vi "ThermoRecDisplay.vi"() -> ()   [LabVIEW 2016]
panel:
  out "SW OPC Error":bool
  out "SS OPC Error":bool
  out "SW ThermoRec Information":string
  out "SS ThermoRec Information":string
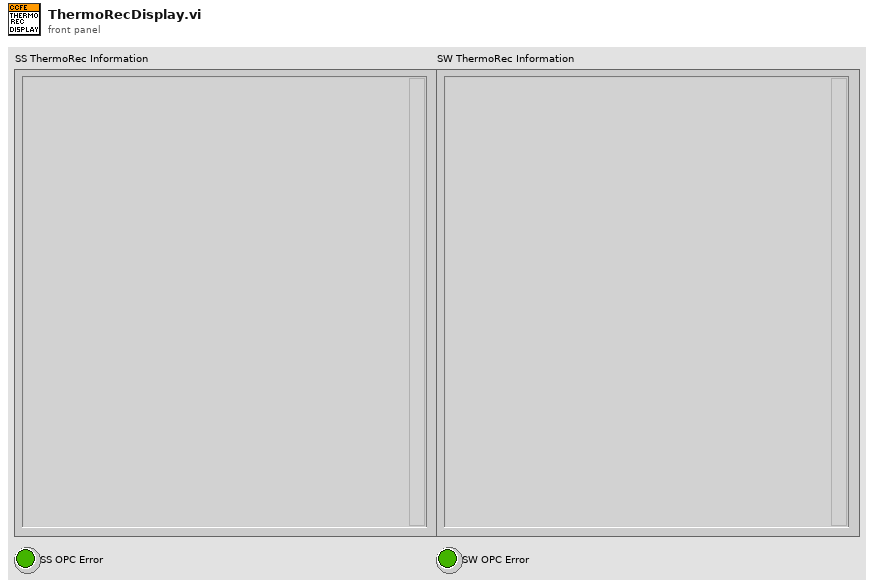
[diagram p1: front panel]
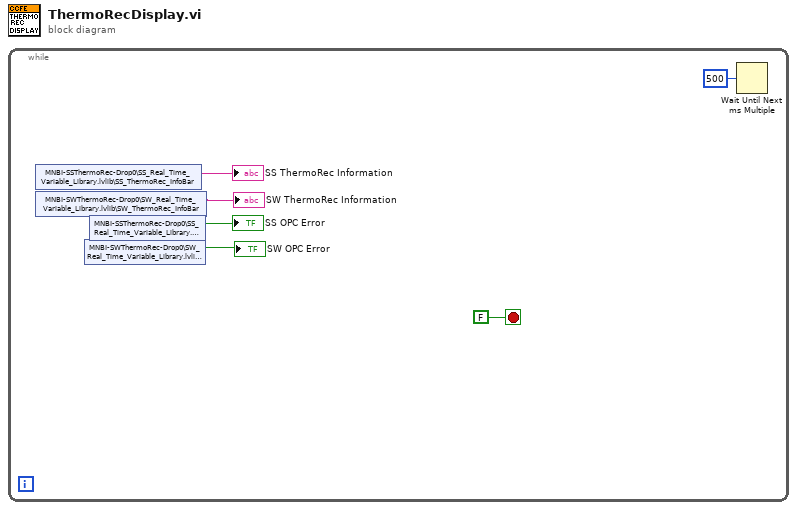
[diagram p0: block diagram]
diagram:
  n1 = while {
    stop <- FALSE stop-if-true
    n2 = shared-variable "MNBI-SSThermoRec-Drop0\\SS_Real_Time_Variable_Library.lvlib\\SS_ThermoRec_InfoBar"() -> (→"SS ThermoRec Information":string)  [unwired: 1 in, 1 out]
    n3 = shared-variable "MNBI-SWThermoRec-Drop0\\SW_Real_Time_Variable_Library.lvlib\\SW_ThermoRec_InfoBar"() -> (→"SW ThermoRec Information":string)  [unwired: 1 in, 1 out]
    n4 = shared-variable "MNBI-SWThermoRec-Drop0\\SW_Real_Time_Variable_Library.lvlib\\SW_OPC_Error"() -> (→"SW OPC Error":bool)  [unwired: 1 in, 1 out]
    n5 = shared-variable "MNBI-SSThermoRec-Drop0\\SS_Real_Time_Variable_Library.lvlib\\SS_OPC_Error"() -> (→"SS OPC Error":bool)  [unwired: 1 in, 1 out]
    n6 = Wait Until Next ms Multiple(millisecond multiple=u32 500) -> ()  [unwired: 1 out]
  }
